vi "User.GetExisting.vi"(1 "Users in":T1[](array[typedef])) -> (0 "Users out":T1[](array[typedef]))   [LabVIEW 2013]
uses:
  User.Info.ctl
  User.Level.ctl
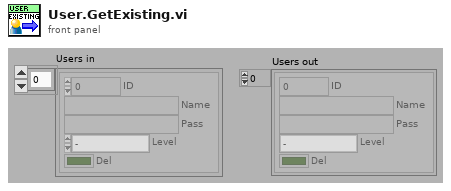
[diagram p1: front panel]
types:
  T1 = typedef "User.Info.ctl" = cluster{"ID":i32, "Name":string, "Pass":string, "Level":T2, "Del":bool}
  T2 = typedef "User.Level.ctl" = enum16{"-", "Operator", "Technician", "Administrator"}
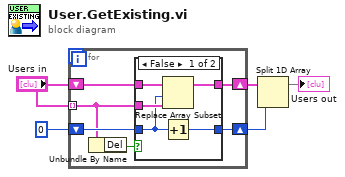
[diagram p0: block diagram]
diagram:
  n1 = for {
    tunnel: "Users in" -> [w7] mode=indexing
    shift-right: [w10] -> w3
    shift-left: "Users in" -> [w11]
    shift-right: [w8] -> w2
    shift-left: 0 -> [w9]
    n2 = Unbundle By Name(w7) -> ("Del"=w6:bool)
    n3 = case shown="False" w6 {
      tunnel: w11 -> [w16 w18]
      tunnel: [w15 w18] -> w10
      tunnel: w7 -> [w14 _]
      tunnel: w9 -> [w13 w17]
      tunnel: [w12 w17] -> w8
      frame False {
        n4 = Replace Array Subset(array=w16, new element=w14, index=w13) -> (w15:T1[])
        n5 = Increment(x=w13) -> (x+1=w12:i32)
      }
      frame True {
      }
    }
  }
  n6 = Split 1D Array(array=w3, index=w2) -> (first subarray=→"Users out":T1[])  [unwired: 1 out]
